vi "Delete Queue.vi"(8 "error in (no error)":errorcluster, 11 "SQS":refnum<class "Queue.lvclass">) -> (0 "error out":errorcluster)   [LabVIEW 2015, in "NI_AWS_SQS.lvlib" / "Queue.lvclass"]
doc: "Deletes the queue specified by the QueueUrl, even if the queue is empty. If the specified queue doesn't exist, Amazon SQS returns a successful response.\n\nImportant\nBe careful with the Delete Queue action: When you delete a queue, any messages in the queue are no longer available.\nWhen you delete a queue, the deletion process takes up to 60 seconds. Requests you send involving that queue during the 60 seconds might succeed. For example, a Send Message request might succeed, but after 60 seconds the queue and the message you sent no longer exist.\n\nWhen you delete a queue, you must wait at least 60 seconds before creating a queue with the same name."
uses:
  Queue.lvclass
  Core/HTTP Request/Request Options.ctl
  Core/HTTP Request/Name Value Pair.ctl
  Core/HTTP Request/Region handling.ctl
  Core/HTTP Request/URL formatting.ctl
  Queue.lvclass/Queue.ctl
  Read Account Number.vi
  Read Name.vi
  Core/HTTP Request/HTTP Request.lvclass
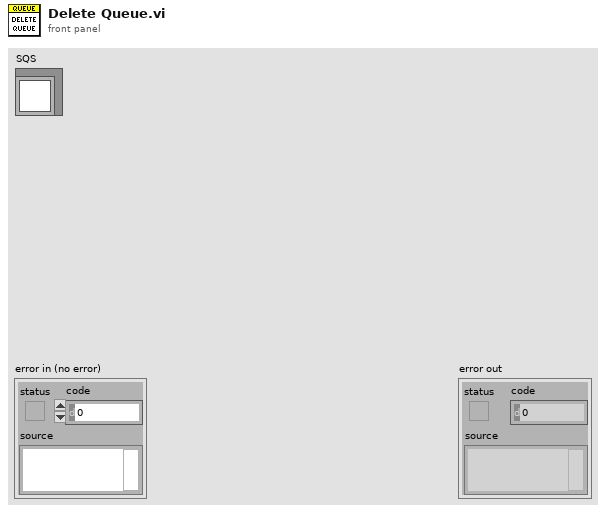
[diagram p1: front panel]
types:
  T1 = typedef "NI_AWS_Core.lvlib/HTTP Request.lvclass/Name Value Pair.ctl" = cluster{"name":string, "value":string}
  T2 = typedef "NI_AWS_Core.lvlib/HTTP Request.lvclass/Request Options.ctl" = cluster{"request headers":T1[], "request parameters":T1[], "request body":string, "region handling":T3, "URL formatting":T4}
  T3 = typedef "NI_AWS_Core.lvlib/HTTP Request.lvclass/Region handling.ctl" = enum16{"use region everywhere", "use region (authentication only)", "use region (URL only)", "ignore region everwhere"}
  T4 = typedef "NI_AWS_Core.lvlib/HTTP Request.lvclass/URL formatting.ctl" = enum16{"region-", "region."}
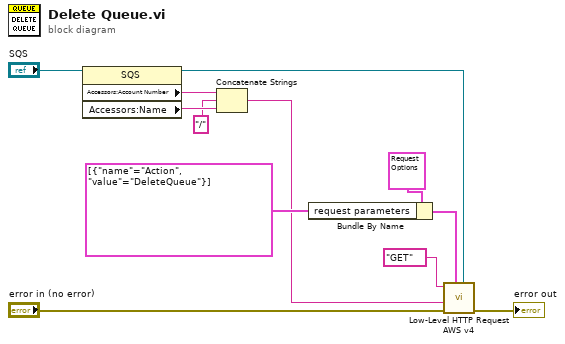
[diagram p0: block diagram]
diagram:
  n1 = property class="SQS"(reference="SQS") -> (reference out=w2:refnum<class "Queue.lvclass">, "Accessors:Account Number"=w6:string, "Accessors:Name"=w5:string)  [unwired: 1 in, 1 out]
  n2 = Concatenate Strings(w6, "/", w5) -> (w1:string)
  n3 = Bundle By Name(cluster=T2 {"request headers"=[], "request parameters"=[{"name"="Action", "value"="ListQueues"}], "request body"="", "region handling"=enum."use region everywhere", "URL formatting"=enum."region."} ("Request Options"), "request parameters"=T1[] [{"name"="Action", "value"="DeleteQueue"}]) -> (w10:T2)
  n4 = call "Low-Level HTTP Request AWS v4.vi"("AWS Core"=w2, "Request Options"=w10, "error in (no error)"="error in (no error)", "URL Suffix"=w1, "HTTP-Verb"="GET") -> ("error out"=→"error out":errorcluster)  [unwired: 4 in, 2 out]
